vi "Upgrade Package.vi"(8 "error in":errorcluster, 11 "package name":string) -> (0 "error out":errorcluster, 1 "previously installed version":string, 2 "currently installed version":string, 3 "package name out":string)   [LabVIEW 2014, in "NIPM_API.lvlib"]
doc: "Upgrades an installed package to the latest available version that is higher than the currently installed version.\n\nNote: This VI will launch a Windows dialog asking for permission to run and requires the user to have admin rights.\n\nINPUT(s)\n<B>Package name</B>: Specifies the package to upgrade.\n\nOUTPUT(s)\n<B>Package name</B>: Outputs the package name.\n\n<B>Currently installed version</B>: Outputs the currently installed version of the specified package after this VI tries to upgrade the package.\n\n<B>Previously installed version</B>: Outputs the version (if any) of the specified package before this VI tries to upgrade the package."
uses:
  NIPM_API.lvlib
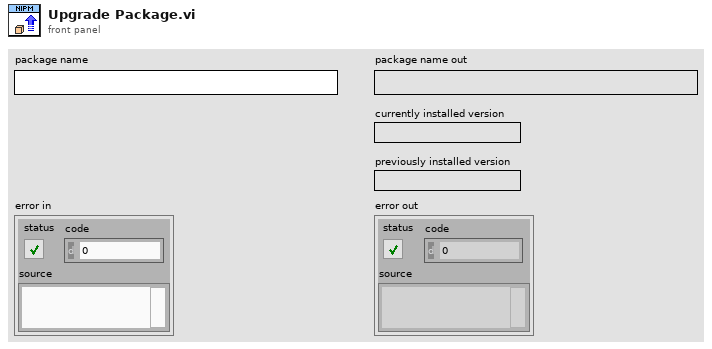
[diagram p1: front panel]
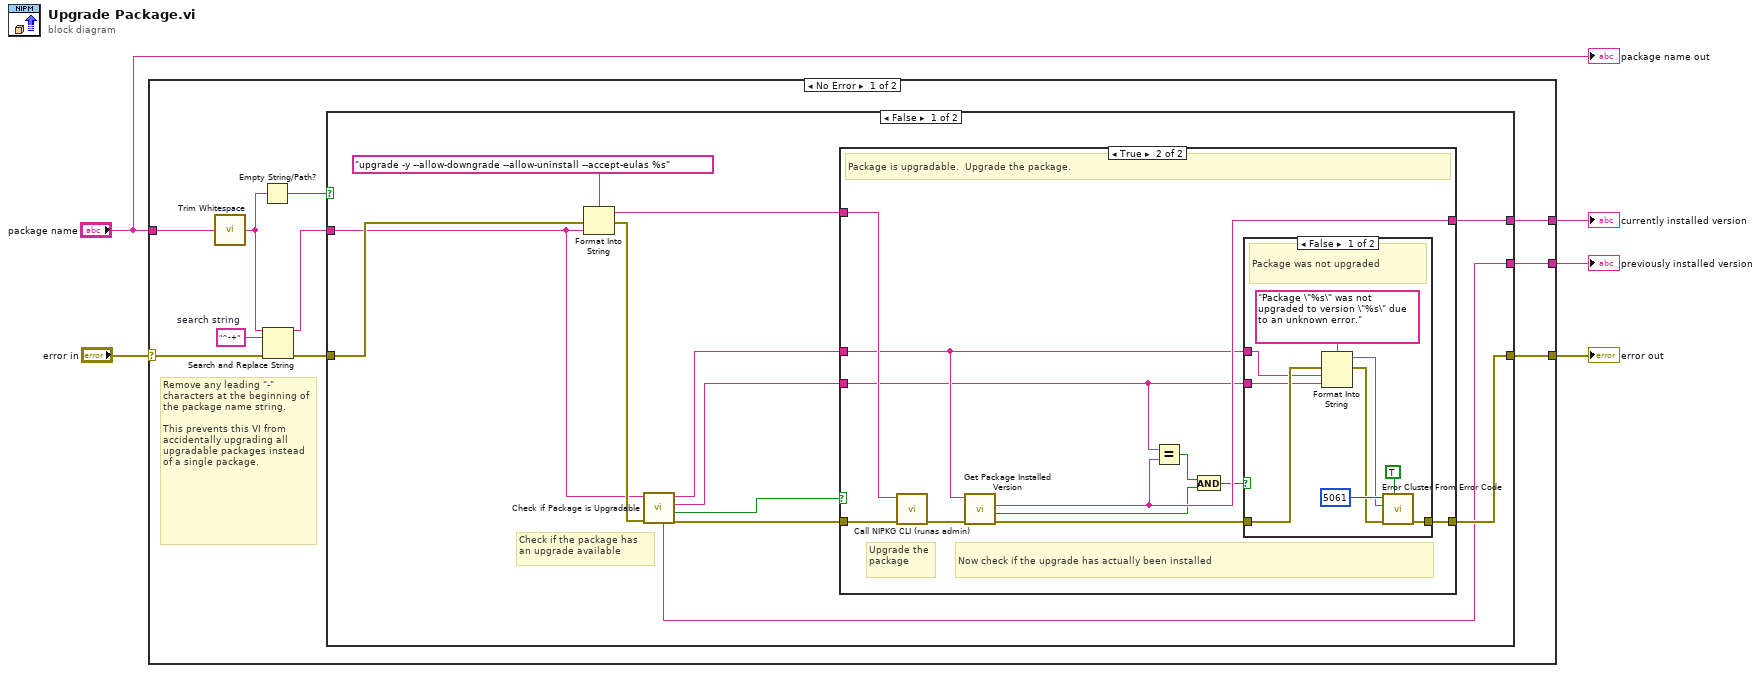
[diagram p0: block diagram]
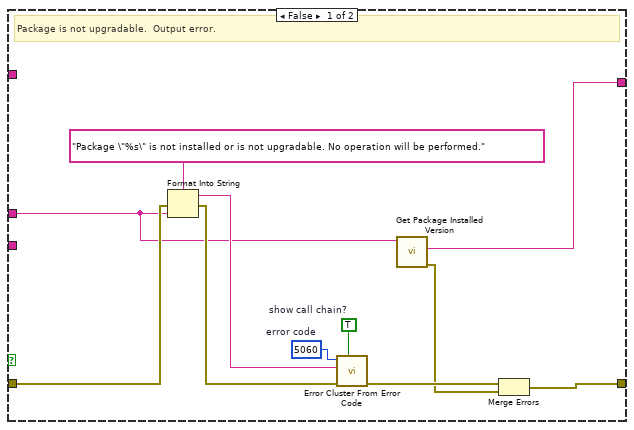
[diagram p2: hidden frame]
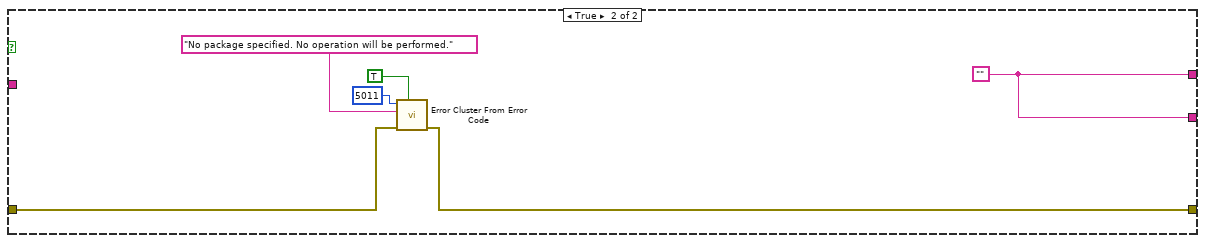
[diagram p4: hidden frame]
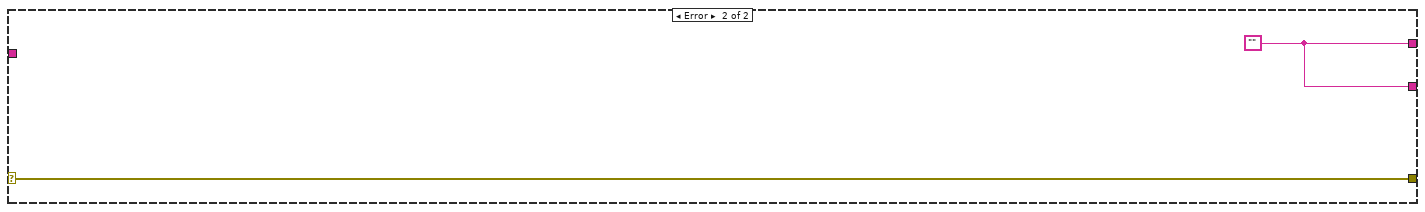
[diagram p5: hidden frame]
diagram:
  n1 = case shown="No Error" "error in" {
    selector: "error in" -> [w11 w67]
    tunnel: [w15 w67] -> w4
    tunnel: "package name" -> [w13 _]
    tunnel: [w14 w66] -> w2
    tunnel: [w6 w66] -> w1
    frame No Error {
      w9 = "^-+"  # search string
      # "Remove any leading \"-\" characters at the beginning of the package name string. \n\nThis prevents this VI from accidentally upgrading all upgradable packages instead of a single package."
      n2 = call <vilib>:"Trim Whitespace.vi"("string"=w13) -> ("trimmed string"=w8:string)  [unwired: 1 in]
      n3 = Empty String/Path?(string/path=w8) -> (empty?=w12:bool)
      n4 = Search and Replace String(input string=w8, search string=w9, error in=w11) -> (result string=w7:string, error out=w10:errorcluster)  [unwired: 5 in, 2 out]
      n5 = case shown="False" w12 {
        tunnel: w10 -> [w26 w62]
        tunnel: [w24 w61] -> w15
        tunnel: [w23 w60] -> w14
        tunnel: w7 -> [w19 _]
        tunnel: [w16 w60] -> w6
        frame False {
          # "Check if the package has an upgrade available"
          n6 = Format Into String(format string="upgrade -y --allow-downgrade --allow-uninstall --accept-eulas %s", error in=w26, w19) -> (resulting string=w25:string, error out=w21:errorcluster)  [unwired: 1 in]
          n7 = call "Check if Package is Upgradable.vi"("error in"=w21, "package name"=w19) -> ("error out"=w20:errorcluster, "upgradable?"=w17:bool, "version to upgrade to"=w18:string, "package name out"=w22:string, "currently installed version"=w16:string)  [unwired: 5 in]
          n8 = case shown="True" w17 {
            tunnel: w25 -> [_ w49]
            tunnel: [w30 w48] -> w24
            tunnel: [w28 w47] -> w23
            tunnel: w22 -> [w31 w41]
            tunnel: w20 -> [w37 w40]
            tunnel: w18 -> [_ w39]
            frame False {
              w33 = TRUE  # show call chain?
              w34 = 5060  # error code
              # "Package is not upgradable.  Output error."
              n9 = Format Into String(format string="Package \"%s\" is not installed or is not upgradable. No operation will be performed.", error in=w37, w31) -> (resulting string=w35:string, error out=w36:errorcluster)  [unwired: 1 in]
              n10 = call <vilib>:"Error Cluster From Error Code.vi"("show call chain? (False)"=w33, "error in (no error)"=w36, "error message (\"\")"=w35, "error code (0)"=w34) -> ("error out"=w32:errorcluster)  [unwired: 5 in]
              n11 = call "Get Package Installed Version.vi"("package name"=w31) -> ("error out"=w29:errorcluster, "installed version"=w28:string)  [unwired: 7 in, 2 out]
              n12 = Merge Errors(w32, w29) -> (w30:errorcluster)
            }
            frame True {
              # "Upgrade the package"
              # "Now check if the upgrade has actually been installed"
              # "Package is upgradable.  Upgrade the package."
              n13 = call "Call NIPKG CLI (runas admin).vi"("error in (no error)"=w40, "command"=w49) -> ("error out"=w46:errorcluster)  [unwired: 9 in]
              n14 = call "Get Package Installed Version.vi"("error in"=w46, "package name"=w41) -> ("error out"=w45:errorcluster, "installed?"=w42:bool, "installed version"=w47:string)  [unwired: 6 in, 1 out]
              n15 = Equal?(x=w39, y=w47) -> (x = y?=w44:bool)
              n16 = And(x=w44, y=w42) -> (x .and. y?=w43:bool)
              n17 = case shown="False" w43 {
                tunnel: w45 -> [w53 w59]
                tunnel: [w56 w59] -> w48
                tunnel: w41 -> [w52 _]
                tunnel: w39 -> [w50 _]
                frame False {
                  # "Package was not upgraded"
                  n18 = Format Into String(format string="Package \"%s\" was not upgraded to version \"%s\" due to an unknown error.", error in=w53, w52, w50) -> (resulting string=w51:string, error out=w54:errorcluster)  [unwired: 1 in]
                  n19 = call <vilib>:"Error Cluster From Error Code.vi"("show call chain? (False)"=TRUE, "error in (no error)"=w54, "error message (\"\")"=w51, "error code (0)"=5061) -> ("error out"=w56:errorcluster)  [unwired: 5 in]
                }
                frame True {
                  # "Upgrade has installed successfully."
                }
              }
            }
          }
        }
        frame True {
          w60 = ""
          n20 = call <vilib>:"Error Cluster From Error Code.vi"("show call chain? (False)"=TRUE, "error in (no error)"=w62, "error message (\"\")"="No package specified. No operation will be performed.", "error code (0)"=5011) -> ("error out"=w61:errorcluster)  [unwired: 5 in]
        }
      }
    }
    frame Error {
      w66 = "" ("standard output")
    }
  }
  "error out" <- w4
  "currently installed version" <- w2
  "previously installed version" <- w1
  "package name out" <- "package name"
